vi "GetMeasurements (Switch GIPB).vi"() -> ()   [LabVIEW 2015]
uses:
  <vilib>/Utility/file.llb/Write Delimited Spreadsheet (DBL).vi
  <instrlib>/Keithley 2182/Keithley 2182.lvlib
panel:
  in  "DVM resource name":refnum<visa-resource-name>="GPIB0::17::INSTR"
  out "?":dbl=198.8220615594723
  in  "Switched GIPB?":bool
  out "Ready To Switch GIPB":bool
  out "Complete?":bool
  in  "+B Field Added?":bool
  out "Ready To Change Field":bool
  in  "-B Field Added? 2":bool
  out "Ready To Change Field":bool
  in  "Set Current (nA)":dbl=1000.0 format="%.3f"
  in  "Voltage Measurement Path?":path=path "C:/Users/oodumosu/Desktop/KO StartUp/Test/ITO_Test0.txt"
  in  "Current Source GPIB Address":string="23"
  # "minutes"
  # "SetUp DVM"
  # "2:"
  # "1:"
  # "SetUp Current Source"
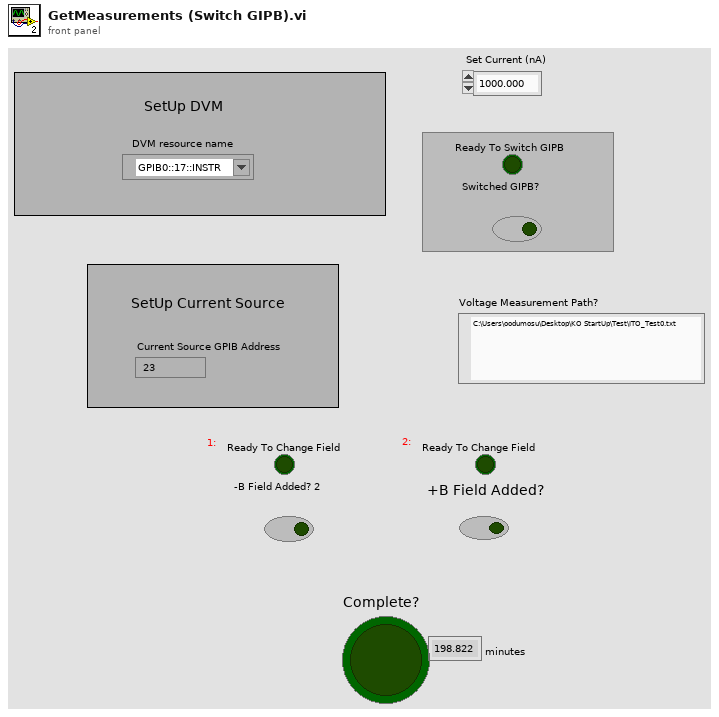
[diagram p1: front panel]
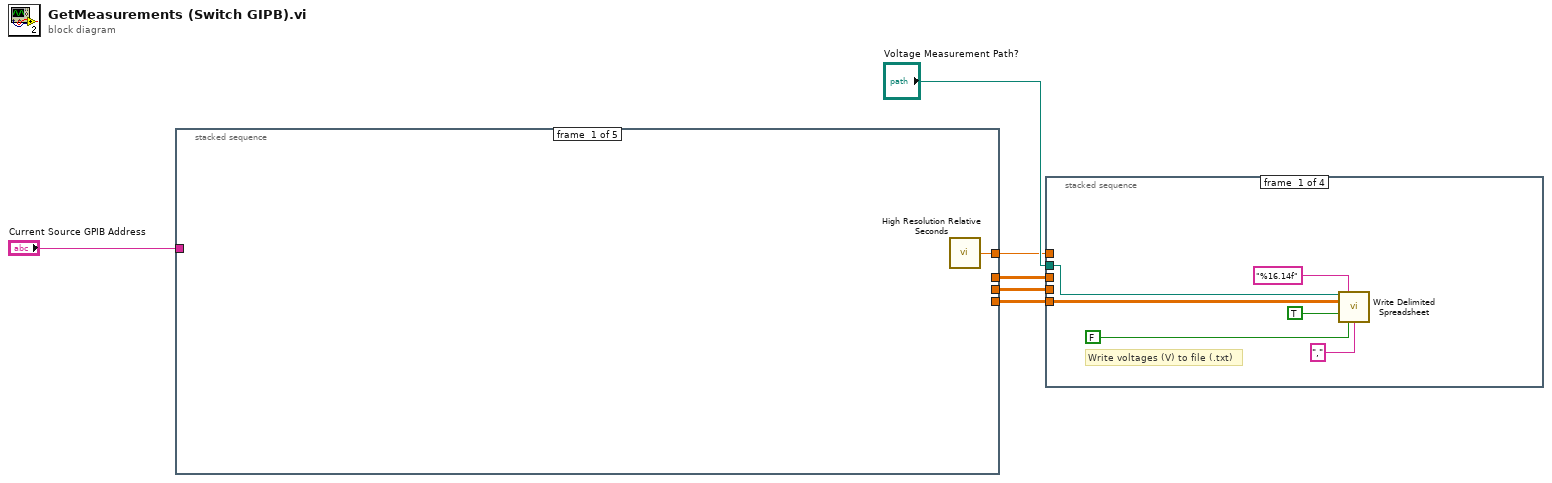
[diagram p0: block diagram]
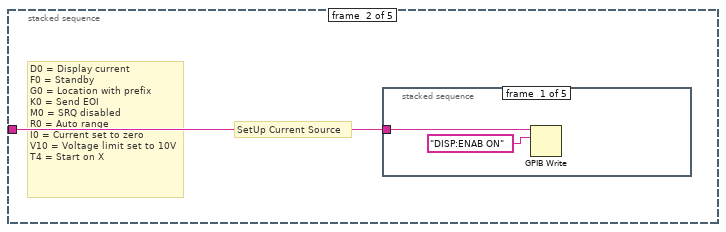
[diagram p2: hidden frame]
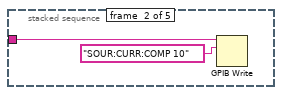
[diagram p3: hidden frame]
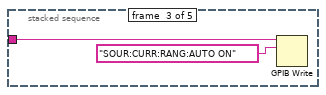
[diagram p4: hidden frame]
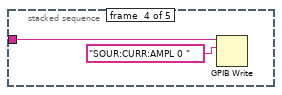
[diagram p5: hidden frame]
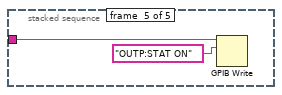
[diagram p6: hidden frame]
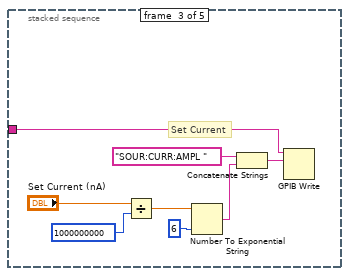
[diagram p7: hidden frame]
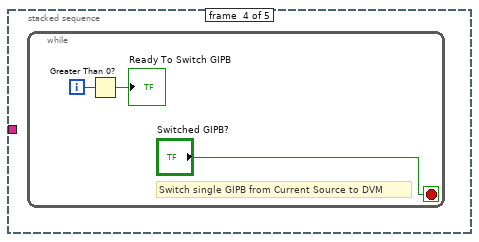
[diagram p8: hidden frame]
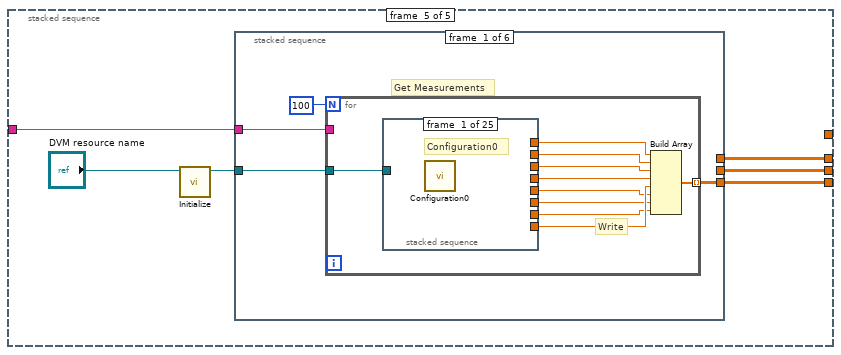
[diagram p9: hidden frame]
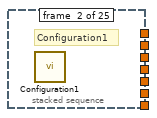
[diagram p10: hidden frame]
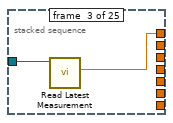
[diagram p11: hidden frame]
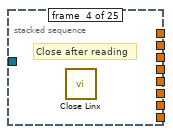
[diagram p12: hidden frame]
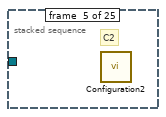
[diagram p13: hidden frame]
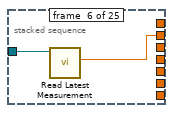
[diagram p14: hidden frame]
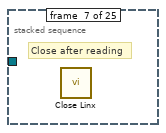
[diagram p15: hidden frame]
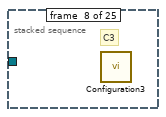
[diagram p16: hidden frame]
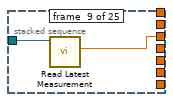
[diagram p17: hidden frame]
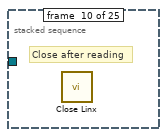
[diagram p18: hidden frame]
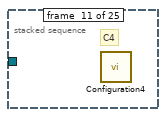
[diagram p19: hidden frame]
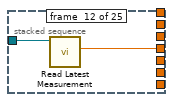
[diagram p20: hidden frame]
diagram:
  n1 = stacked-sequence {
    tunnel: "Current Source GPIB Address" -> [_ w8 w20 _ w33]
    tunnel: [w7 _ _ _ _] -> w4
    tunnel: [_ _ _ _ w32] -> w3
    tunnel: [_ _ _ _ w31] -> w2
    tunnel: [_ _ _ _ w30] -> w1
    frame #0 {
      n2 = call <vilib>:"High Resolution Relative Seconds.vi"() -> ("relative seconds"=w7:dbl)
    }
    frame #1 {
      # "SetUp Current Source"
      # "D0 = Display current\nF0 = Standby\nG0 = Location with prefix\nK0 = Send EOI\nM0 = SRQ disabled\nR0 = Auto range\nI0 = Current set to zero\nV10 = Voltage limit set to 10V\nT4 = Start on X"
      n3 = stacked-sequence {
        tunnel: w8 -> [w9 w11 w13 w15 w17]
        frame #0 {
          n4 = GPIB Write(0:w9, 1:"DISP:ENAB ON") -> ()  [unwired: 3 in, 2 out]
        }
        frame #1 {
          n5 = GPIB Write(0:w11, 1:"SOUR:CURR:COMP 10") -> ()  [unwired: 3 in, 2 out]
        }
        frame #2 {
          n6 = GPIB Write(0:w13, 1:"SOUR:CURR:RANG:AUTO ON") -> ()  [unwired: 3 in, 2 out]
        }
        frame #3 {
          n7 = GPIB Write(0:w15, 1:"SOUR:CURR:AMPL 0 ") -> ()  [unwired: 3 in, 2 out]
        }
        frame #4 {
          n8 = GPIB Write(0:w17, 1:"OUTP:STAT ON") -> ()  [unwired: 3 in, 2 out]
        }
      }
    }
    frame #2 {
      # "Set Current"
      n9 = Divide(x="Set Current (nA)", y=1000000000) -> (x/y=w22:dbl)
      n10 = Number To Exponential String(number=w22, precision (6)=6) -> (E-format string=w23:string)  [unwired: 2 in]
      n11 = Concatenate Strings("SOUR:CURR:AMPL ", w23) -> (w25:string)
      n12 = GPIB Write(0:w20, 1:w25) -> ()  [unwired: 3 in, 2 out]
    }
    frame #3 {
      n13 = while {
        i -> [w28]
        stop <- "Switched GIPB?" stop-if-true
        # "Switch single GIPB from Current Source to DVM"
        n14 = Greater Than 0?(x=w28) -> (x > 0?=→"Ready To Switch GIPB":bool)
      }
    }
    frame #4 {
      n15 = call <instrlib>:"Initialize.vi"("VISA resource name"="DVM resource name") -> ("VISA resource name out"=w34:refnum<visa-resource-name>)  [unwired: 9 in, 1 out]
      n16 = stacked-sequence {
        tunnel: w33 -> [w38 _ _ _ _ _]
        tunnel: [w37 _ _ _ _ _] -> w32
        tunnel: [_ _ w70 _ _ _] -> w31
        tunnel: [_ _ _ _ w91 _] -> w30
        tunnel: w34 -> [w36 _ w69 _ w89 _]
        frame #0 {
          # "Get Measurements"
          n17 = for {
            N: 100 -> [_]
            tunnel: [w49] -> w37 mode=indexing
            tunnel: w38 -> [_]
            tunnel: w36 -> [w48]
            # "Write"
            n18 = stacked-sequence {
              tunnel: w48 -> [_ _ w51 _ _ w53 _ _ w55 _ _ w57 _ _ w59 _ _ w61 _ _ w63 _ _ w65 _]
              tunnel: [_ _ w50 _ _ _ _ _ _ _ _ _ _ _ _ _ _ _ _ _ _ _ _ _ _] -> w47
              tunnel: [_ _ _ _ _ w52 _ _ _ _ _ _ _ _ _ _ _ _ _ _ _ _ _ _ _] -> w46
              tunnel: [_ _ _ _ _ _ _ _ w54 _ _ _ _ _ _ _ _ _ _ _ _ _ _ _ _] -> w45
              tunnel: [_ _ _ _ _ _ _ _ _ _ _ w56 _ _ _ _ _ _ _ _ _ _ _ _ _] -> w44
              tunnel: [_ _ _ _ _ _ _ _ _ _ _ _ _ _ w58 _ _ _ _ _ _ _ _ _ _] -> w43
              tunnel: [_ _ _ _ _ _ _ _ _ _ _ _ _ _ _ _ _ w60 _ _ _ _ _ _ _] -> w42
              tunnel: [_ _ _ _ _ _ _ _ _ _ _ _ _ _ _ _ _ _ _ _ w62 _ _ _ _] -> w41
              tunnel: [_ _ _ _ _ _ _ _ _ _ _ _ _ _ _ _ _ _ _ _ _ _ _ w64 _] -> w40
              frame #0 {
                # "Configuration0"
                n19 = call "Configuration0.vi"() -> ()  [unwired: 12 in]
              }
              frame #1 {
                # "Configuration1"
                n20 = call "Configuration1.vi"() -> ()  [unwired: 12 in]
              }
              frame #2 {
                n21 = call <instrlib>:"Read Latest Measurement.vi"("VISA resource name"=w51) -> ("Measurement"=w50:dbl)  [unwired: 7 in, 3 out]
              }
              frame #3 {
                # "Close after reading"
                n22 = call "Close Linx.vi"() -> ()  [unwired: 12 in]
              }
              frame #4 {
                # "C2"
                n23 = call "Configuration2.vi"() -> ()  [unwired: 12 in]
              }
              frame #5 {
                n24 = call <instrlib>:"Read Latest Measurement.vi"("VISA resource name"=w53) -> ("Measurement"=w52:dbl)  [unwired: 7 in, 3 out]
              }
              frame #6 {
                # "Close after reading"
                n25 = call "Close Linx.vi"() -> ()  [unwired: 12 in]
              }
              frame #7 {
                # "C3"
                n26 = call "Configuration3.vi"() -> ()  [unwired: 12 in]
              }
              frame #8 {
                n27 = call <instrlib>:"Read Latest Measurement.vi"("VISA resource name"=w55) -> ("Measurement"=w54:dbl)  [unwired: 7 in, 3 out]
              }
              frame #9 {
                # "Close after reading"
                n28 = call "Close Linx.vi"() -> ()  [unwired: 12 in]
              }
              frame #10 {
                # "C4"
                n29 = call "Configuration4.vi"() -> ()  [unwired: 12 in]
              }
              frame #11 {
                n30 = call <instrlib>:"Read Latest Measurement.vi"("VISA resource name"=w57) -> ("Measurement"=w56:dbl)  [unwired: 7 in, 3 out]
              }
              frame #12 {
                # "Close after reading"
                n31 = call "Close Linx.vi"() -> ()  [unwired: 12 in]
              }
              frame #13 {
                # "C5"
                n32 = call "Configuration5.vi"() -> ()  [unwired: 12 in]
              }
              frame #14 {
                n33 = call <instrlib>:"Read Latest Measurement.vi"("VISA resource name"=w59) -> ("Measurement"=w58:dbl)  [unwired: 7 in, 3 out]
              }
              frame #15 {
                # "Close after reading"
                n34 = call "Close Linx.vi"() -> ()  [unwired: 12 in]
              }
              frame #16 {
                # "C6"
                n35 = call "Configuration6.vi"() -> ()  [unwired: 12 in]
              }
              frame #17 {
                n36 = call <instrlib>:"Read Latest Measurement.vi"("VISA resource name"=w61) -> ("Measurement"=w60:dbl)  [unwired: 7 in, 3 out]
              }
              frame #18 {
                # "Close after reading"
                n37 = call "Close Linx.vi"() -> ()  [unwired: 12 in]
              }
              frame #19 {
                # "C7"
                n38 = call "Configuration7.vi"() -> ()  [unwired: 12 in]
              }
              frame #20 {
                n39 = call <instrlib>:"Read Latest Measurement.vi"("VISA resource name"=w63) -> ("Measurement"=w62:dbl)  [unwired: 7 in, 3 out]
              }
              frame #21 {
                # "Close after reading"
                n40 = call "Close Linx.vi"() -> ()  [unwired: 12 in]
              }
              frame #22 {
                # "C8"
                n41 = call "Configuration8.vi"() -> ()  [unwired: 12 in]
              }
              frame #23 {
                n42 = call <instrlib>:"Read Latest Measurement.vi"("VISA resource name"=w65) -> ("Measurement"=w64:dbl)  [unwired: 7 in, 3 out]
              }
              frame #24 {
                # "Close after reading"
                n43 = call "Close Linx.vi"() -> ()  [unwired: 12 in]
              }
            }
            n44 = Build Array(w47, w46, w45, w44, w43, w42, w41, w40) -> (w49:dbl[])
          }
        }
        frame #1 {
          n45 = while {
            i -> [w67]
            stop <- "-B Field Added? 2" stop-if-true
            # "Add -B field"
            n46 = Greater Than 0?(x=w67) -> (x > 0?=→"Ready To Change Field":bool)
          }
        }
        frame #2 {
          n47 = for {
            N: 100 -> [_]
            tunnel: w69 -> [w77]
            tunnel: [w76] -> w70 mode=indexing
            n48 = stacked-sequence {
              tunnel: w77 -> [_ _ w79 _ _ w81 _ _ w83 _ _ w85 _]
              tunnel: [_ _ w78 _ _ _ _ _ _ _ _ _ _] -> w75
              tunnel: [_ _ _ _ _ w80 _ _ _ _ _ _ _] -> w74
              tunnel: [_ _ _ _ _ _ _ _ w82 _ _ _ _] -> w73
              tunnel: [_ _ _ _ _ _ _ _ _ _ _ w84 _] -> w72
              frame #0 {
                # "Reset"
                n49 = call "Configuration0.vi"() -> ()  [unwired: 12 in]
              }
              frame #1 {
                # "C9"
                n50 = call "Configuration9.vi"() -> ()  [unwired: 12 in]
              }
              frame #2 {
                n51 = call <instrlib>:"Read Latest Measurement.vi"("VISA resource name"=w79) -> ("Measurement"=w78:dbl)  [unwired: 7 in, 3 out]
              }
              frame #3 {
                # "Close after reading"
                n52 = call "Close Linx.vi"() -> ()  [unwired: 12 in]
              }
              frame #4 {
                # "C10"
                n53 = call "Configuration10.vi"() -> ()  [unwired: 12 in]
              }
              frame #5 {
                n54 = call <instrlib>:"Read Latest Measurement.vi"("VISA resource name"=w81) -> ("Measurement"=w80:dbl)  [unwired: 7 in, 3 out]
              }
              frame #6 {
                # "Close after reading"
                n55 = call "Close Linx.vi"() -> ()  [unwired: 12 in]
              }
              frame #7 {
                # "C11"
                n56 = call "Configuration11.vi"() -> ()  [unwired: 12 in]
              }
              frame #8 {
                n57 = call <instrlib>:"Read Latest Measurement.vi"("VISA resource name"=w83) -> ("Measurement"=w82:dbl)  [unwired: 7 in, 3 out]
              }
              frame #9 {
                # "Close after reading"
                n58 = call "Close Linx.vi"() -> ()  [unwired: 12 in]
              }
              frame #10 {
                # "C12"
                n59 = call "Configuration12.vi"() -> ()  [unwired: 12 in]
              }
              frame #11 {
                n60 = call <instrlib>:"Read Latest Measurement.vi"("VISA resource name"=w85) -> ("Measurement"=w84:dbl)  [unwired: 7 in, 3 out]
              }
              frame #12 {
                # "Close after reading"
                n61 = call "Close Linx.vi"() -> ()  [unwired: 12 in]
              }
            }
            n62 = Build Array(w75, w74, w73, w72) -> (w76:dbl[])
          }
        }
        frame #3 {
          # "Change to +B Field"
          n63 = while {
            i -> [w86]
            stop <- "+B Field Added?" stop-if-true
            n64 = Greater Than 0?(x=w86) -> (x > 0?=→"Ready To Change Field":bool)
          }
        }
        frame #4 {
          n65 = for {
            N: 100 -> [_]
            tunnel: w89 -> [w97]
            tunnel: [w92] -> w91 mode=indexing
            n66 = stacked-sequence {
              tunnel: w97 -> [_ _ w99 _ _ w101 _ _ w103 _ _ w105 _]
              tunnel: [_ _ w98 _ _ _ _ _ _ _ _ _ _] -> w96
              tunnel: [_ _ _ _ _ w100 _ _ _ _ _ _ _] -> w95
              tunnel: [_ _ _ _ _ _ _ _ w102 _ _ _ _] -> w94
              tunnel: [_ _ _ _ _ _ _ _ _ _ _ w104 _] -> w93
              frame #0 {
                # "Reset"
                n67 = call "Configuration0.vi"() -> ()  [unwired: 12 in]
              }
              frame #1 {
                # "C13"
                n68 = call "Configuration9.vi"() -> ()  [unwired: 12 in]
              }
              frame #2 {
                n69 = call <instrlib>:"Read Latest Measurement.vi"("VISA resource name"=w99) -> ("Measurement"=w98:dbl)  [unwired: 7 in, 3 out]
              }
              frame #3 {
                # "Close after reading"
                n70 = call "Close Linx.vi"() -> ()  [unwired: 12 in]
              }
              frame #4 {
                # "C14"
                n71 = call "Configuration10.vi"() -> ()  [unwired: 12 in]
              }
              frame #5 {
                n72 = call <instrlib>:"Read Latest Measurement.vi"("VISA resource name"=w101) -> ("Measurement"=w100:dbl)  [unwired: 7 in, 3 out]
              }
              frame #6 {
                # "Close after reading"
                n73 = call "Close Linx.vi"() -> ()  [unwired: 12 in]
              }
              frame #7 {
                # "C15"
                n74 = call "Configuration11.vi"() -> ()  [unwired: 12 in]
              }
              frame #8 {
                n75 = call <instrlib>:"Read Latest Measurement.vi"("VISA resource name"=w103) -> ("Measurement"=w102:dbl)  [unwired: 7 in, 3 out]
              }
              frame #9 {
                # "Close after reading"
                n76 = call "Close Linx.vi"() -> ()  [unwired: 12 in]
              }
              frame #10 {
                # "C16"
                n77 = call "Configuration12.vi"() -> ()  [unwired: 12 in]
              }
              frame #11 {
                n78 = call <instrlib>:"Read Latest Measurement.vi"("VISA resource name"=w105) -> ("Measurement"=w104:dbl)  [unwired: 7 in, 3 out]
              }
              frame #12 {
                # "Close after reading"
                n79 = call "Close Linx.vi"() -> ()  [unwired: 12 in]
              }
            }
            n80 = Build Array(w96, w95, w94, w93) -> (w92:dbl[])
          }
        }
        frame #5 {
          "Complete?" <- TRUE
        }
      }
    }
  }
  n81 = stacked-sequence {
    tunnel: "Voltage Measurement Path?" -> [w108 w114 w120 _]
    tunnel: w3 -> [w107 _ _ _]
    tunnel: w2 -> [_ w113 _ _]
    tunnel: w4 -> [_ _ _ w125]
    tunnel: w1 -> [_ _ w119 _]
    frame #0 {
      # "Write voltages (V) to file (.txt)"
      n82 = call-poly <vilib>:"Write Delimited Spreadsheet.vi"("file path (dialog if empty)"=w108, "format (%.3f)"="%16.14f", "2D data"=w107, "append to file? (F)"=TRUE, "transpose? (F)"=FALSE, "delimiter (\\t)"="," ("delimiter (\\t)")) -> ()  [unwired: 8 in, 2 out]
    }
    frame #1 {
      # "Write voltages (V) to file (.txt)"
      n83 = call-poly <vilib>:"Write Delimited Spreadsheet.vi"("file path (dialog if empty)"=w114, "format (%.3f)"="%16.14f", "2D data"=w113, "append to file? (F)"=TRUE, "transpose? (F)"=FALSE, "delimiter (\\t)"="," ("delimiter (\\t)")) -> ()  [unwired: 8 in, 2 out]
    }
    frame #2 {
      n84 = call-poly <vilib>:"Write Delimited Spreadsheet.vi"("file path (dialog if empty)"=w120, "format (%.3f)"="%16.14f", "2D data"=w119, "append to file? (F)"=TRUE, "transpose? (F)"=FALSE, "delimiter (\\t)"="," ("delimiter (\\t)")) -> ()  [unwired: 8 in, 2 out]
    }
    frame #3 {
      # "Calculate and display total run time of program"
      n85 = call <vilib>:"High Resolution Relative Seconds.vi"() -> ("relative seconds"=w129:dbl)
      n86 = Subtract(x=w129, y=w125) -> (x-y=w128:dbl)
      n87 = Divide(x=w128, y=60.0) -> (x/y=→"?":dbl)
    }
  }
